vi "Test_PublishI32_PubBeforeSub_OK.vi"(8 "error in (no error)":errorcluster, 11 "TestMediator In":refnum<class "TestMediator.lvclass">) -> (0 "error out":errorcluster, 3 "TestMediator Out":refnum<class "TestMediator.lvclass">)   [LabVIEW 2017, in "TestMediator.lvclass"]
uses:
  TestMediator.lvclass
  Mediator/Mediator.lvclass
  C:/Program Files (x86)/National Instruments/LabVIEW 2017/vi.lib/ActorFramework/Actor/Actor.lvclass
  IMediator/PublishRequest/PublishRequest.lvclass/PublishRequest.ctl
  Transport/QueueTransport/QueueTransport.lvclass/QueueTransport.ctl
  SubscriptionPolicy/BasicSubscription/BasicSubscription.lvclass/BasicSubscription.ctl
  IMediator/SubscriptionRequest/SubscriptionRequest.lvclass/SubscriptionRequest.ctl
  IMediator/IMediator Messages/Publish Msg/Publish Msg.lvclass/Publish Msg.ctl
  <vilib>/ActorFramework/Message Enqueuer/Message Enqueuer.lvclass/Message Enqueuer.ctl
  IMediator/IMediator Messages/Subscribe Msg/Subscribe Msg.lvclass/Subscribe Msg.ctl
  <vilib>/ActorFramework/Message Enqueuer/Enqueue.vi
  SubscriptionPolicy/BasicSubscription/BasicSubscription.lvclass
  C:/Git/mva-framework/Framework/IMediator/ISubscriptionPolicy/ISubscriptionPolicy.lvclass
  Transport/QueueTransport/QueueTransport.lvclass
  C:/Git/mva-framework/Framework/IMediator/ITransport/ITransport.lvclass
  IMediator/IMediator Messages/Publish Msg/Publish Msg.lvclass
  C:/Program Files (x86)/National Instruments/LabVIEW 2017/vi.lib/ActorFramework/Message/Message.lvclass
  IMediator/IMediator Messages/Subscribe Msg/Subscribe Msg.lvclass
  <vilib>/ActorFramework/Stop Msg/Stop Msg.lvclass
  <vilib>/Utility/error.llb/Error Cluster From Error Code.vi
  <vilib>/ActorFramework/Message Priority Queue/Priority Enqueue.vi
  IMediator/SubscriptionRequest/SubscriptionRequest.lvclass
  IMediator/PublishRequest/PublishRequest.lvclass
  <vilib>/addons/_JKI Toolkits/VI Tester/TestCase.llb/TestCase.lvclass
  <vilib>/ActorFramework/Actor/Actor.lvclass
  IMediator/ISubscriptionPolicy/ISubscriptionPolicy.lvclass
  C:/Program Files (x86)/National Instruments/LabVIEW 2017/vi.lib/addons/_JKI Toolkits/VI Tester/TestCase.llb/TestCase.lvclass
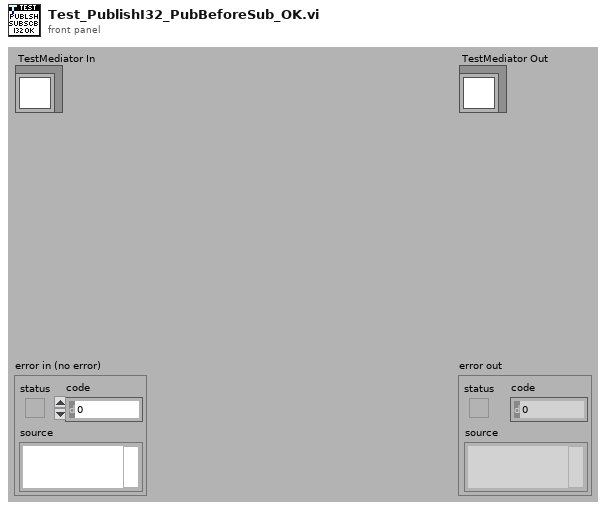
[diagram p1: front panel]
types:
  T1 = typedef "IMediator.lvlib/ISubscriptionPolicy.lvclass/ISubscriptionPolicy Reference.ctl" = refnum<data-value>
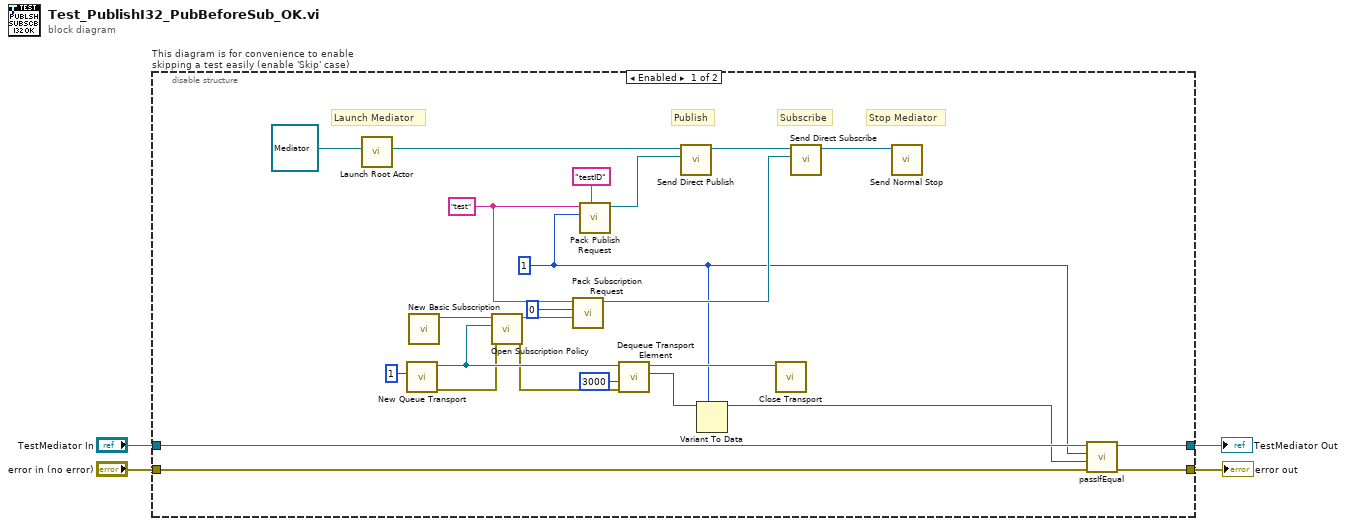
[diagram p0: block diagram]
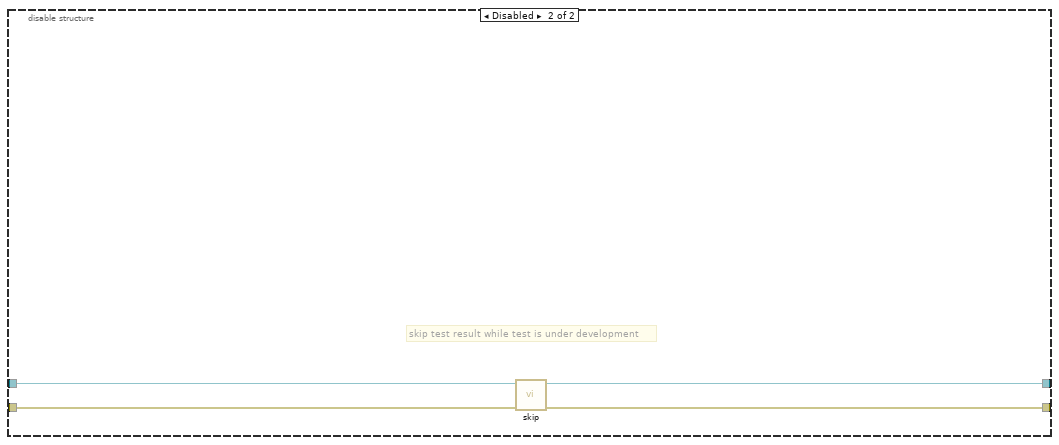
[diagram p2: hidden frame]
diagram:
  n1 = disable-structure "This diagram is for convenience to enable skipping a test easily (enable 'Skip' case)" shown="Enabled" {
    disable-tunnel: "TestMediator In" -> [w28 w32]
    disable-tunnel: [w27 w30] -> w1
    disable-tunnel: [w26 w31] -> w3
    disable-tunnel: "error in (no error)" -> [w25 w29]
    frame Enabled {
      w7 = "test" ("Datum Name")
      w6 = 1
      # "Launch Mediator"
      # "Stop Mediator"
      # "Subscribe"
      # "Publish"
      n2 = call <vilib>:"Launch Root Actor.vi"("Actor"=refnum<class "Mediator.lvclass"> refnum ("Mediator.lvlib:Mediator.lvclass")) -> ("Actor's Enqueuer"=w23:refnum<class "Message Enqueuer.lvclass">)  [unwired: 9 in, 1 out]
      n3 = call "New Queue Transport.vi"("Max Queue Size (-1)"=1) -> ("error out"=w16:errorcluster, "QueueTransport"=w18:refnum<class "QueueTransport.lvclass">)  [unwired: 9 in]
      n4 = call "New Basic Subscription.vi"() -> ("BasicSubscription Out"=w10:refnum<class "BasicSubscription.lvclass">)  [unwired: 11 in]
      n5 = call "Open Subscription Policy.vi"("error in (no error)"=w16, "Transport"=w18, "SubscriptionPolicy"=w10) -> ("error out"=w15:errorcluster, "Subscription Policy"=w9:T1)  [unwired: 7 in]
      n6 = call "Pack Subscription Request.vi"("Subscription Policy"=w9, "Type"=0, "Datum Name"=w7) -> ("SubscriptionRequest"=w22:refnum<class "SubscriptionRequest.lvclass">)  [unwired: 8 in]
      n7 = call "Pack Publish Request.vi"("Publisher ID"="testID", "Data to Publish"=w6, "Datum Name"=w7) -> ("PublishRequest"=w5:refnum<class "PublishRequest.lvclass">)  [unwired: 8 in]
      n8 = call "Dequeue Transport Element.vi"("error in (no error)"=w15, "Timeout In ms (-1)"=3000, "QueueTransport in"=w18) -> ("Data"=w12:variant, "QueueTransport out"=w13:refnum<class "QueueTransport.lvclass">)  [unwired: 5 in, 2 out]
      n9 = call "Send Direct Publish.vi"("PublishRequest"=w5, "Mediator Enqeuer"=w23) -> ("Mediator Enqueuer out"=w21:refnum<class "Message Enqueuer.lvclass">)  [unwired: 8 in, 1 out]
      n10 = Variant To Data(type=w6, Variant=w12) -> (data=w11:i32)  [unwired: 1 in, 1 out]
      n11 = call-dynamic "Close Transport.vi"("QueueTransport in"=w13) -> ()  [unwired: 10 in, 1 out]
      n12 = call "Send Direct Subscribe.vi"("Subscription Request"=w22, "Message Enqueuer"=w21) -> ("Message Enqueuer out"=w14:refnum<class "Message Enqueuer.lvclass">)  [unwired: 8 in, 1 out]
      n13 = call <vilib>:"Send Normal Stop.vi"("Message Enqueuer"=w14) -> ()  [unwired: 10 in, 1 out]
      n14 = call-dynamic "passIfEqual.vi"("error in (no error)"=w25, "y"=w11, "x"=w6, "TestCase in"=w28) -> ("error out"=w26:errorcluster, "TestCase out"=w27:refnum<class "TestMediator.lvclass">)  [unwired: 6 in]
    }
    frame Disabled {
      # "skip test result while test is under development"
      n15 = call <vilib>:"skip.vi"("error in (no error)"=w29, "TestCase in"=w32) -> ("error out"=w31:errorcluster, "TestCase out"=w30:refnum<class "TestMediator.lvclass">)  [unwired: 8 in]
    }
  }
  "error out" <- w3
  "TestMediator Out" <- w1
